vi "check_G1_G2_G3.vi"(0 "current line":string, 3 "error in (no error)":errorcluster) -> (7 "Triggger G1,G2, or G3":bool=TRUE, 9 "error out (no error)":errorcluster)   [LabVIEW 2017]
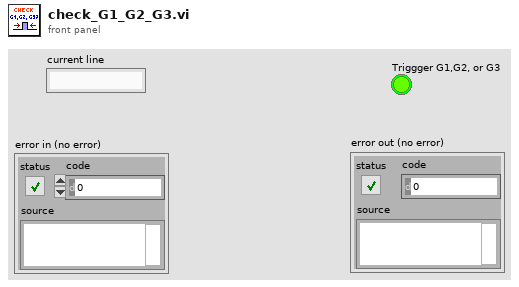
[diagram p1: front panel]
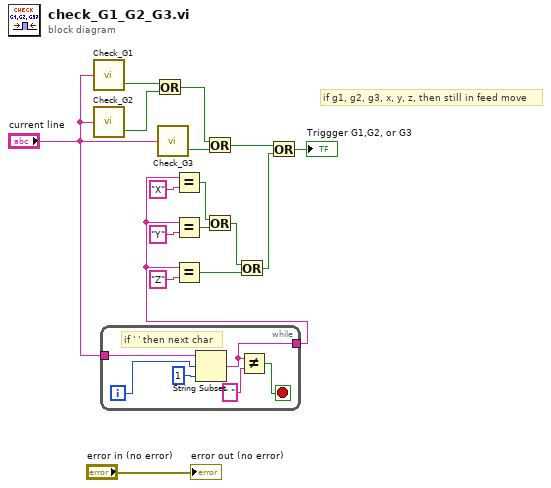
[diagram p0: block diagram]
diagram:
  # "if g1, g2, g3, x, y, z, then still in feed move"
  n1 = call "Check_G1.vi"("trimmed string"="current line") -> ("G1 or G01"=w17:bool)  [unwired: 1 in]
  n2 = call "Check_G2.vi"("trimmed string"="current line") -> ("G2 or G02"=w16:bool)  [unwired: 1 in]
  n3 = while {
    tunnel: "current line" -> [w22]
    tunnel: [w18] -> w1
    i -> [w21]
    stop <- w19 stop-if-true
    # "if ' ' then next char"
    n4 = String Subset(string=w22, offset (0)=w21, length (rest)=1 ("length (rest)")) -> (substring=w18:string)
    n5 = Not Equal?(x=w18, y=" ") -> (x != y?=w19:bool)
  }
  n6 = Or(x=w17, y=w16) -> (x .or. y?=w14:bool)
  n7 = call "Check_G3.vi"("trimmed string"="current line") -> ("G2 or G02"=w15:bool)  [unwired: 1 in]
  n8 = Equal?(x=w1, y="X" ("current line")) -> (x = y?=w9:bool)
  n9 = Equal?(x=w1, y="Y" ("current line")) -> (x = y?=w8:bool)
  n10 = Equal?(x=w1, y="Z" ("current line")) -> (x = y?=w6:bool)
  n11 = Or(x=w14, y=w15) -> (x .or. y?=w4:bool)
  n12 = Or(x=w9, y=w8) -> (x .or. y?=w7:bool)
  n13 = Or(x=w7, y=w6) -> (x .or. y?=w5:bool)
  n14 = Or(x=w4, y=w5) -> (x .or. y?=→"Triggger G1,G2, or G3":bool)
  "error out (no error)" <- "error in (no error)"
